vi "20211022_HW04.vi"() -> ()   [LabVIEW 2019]
panel:
  in  "Calc":bool
  out "Sum":dbl=1.0
  in  "N6":dbl
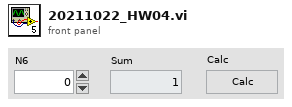
[diagram p1: front panel]
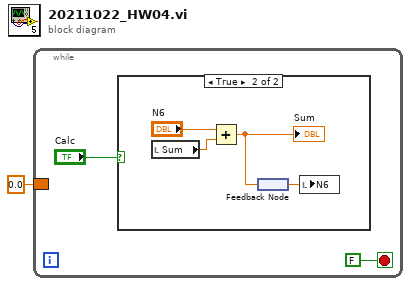
[diagram p0: block diagram]
diagram:
  n1 = while {
    border: 0.0 -> [_]
    stop <- FALSE stop-if-true
    n2 = case shown="True" "Calc" {
      frame False {
      }
      frame True {
        n3 = local read "Sum"() -> (w7:dbl)
        n4 = Add(x="N6", y=w7) -> (x+y=w5:dbl)
        "Sum" <- w5
        n5 = feedback #1() -> (w4:dbl)
        n6 = feedback-in #1(w5) -> ()
        n7 = local write "N6"(w4) -> ()
      }
    }
  }
